vi "Comm_WriteRead.vi"(8 "error in (no error)":errorcluster, 9 "Code":string, 10 "Console In":string, 11 "Python":T1) -> (0 "error out":errorcluster, 2 "Console":string, 3 "Python":T1)   [LabVIEW 2022 SP3]
uses:
  PythonCtrl.ctl
  Processors.ctl
  <vilib>/Utility/error.llb/Trim Whitespace One-Sided.vi
panel:
  out "File sent":string[](array[string])
  out "Array":u32[](array[numeric])
  out "replies":string[](array[string])
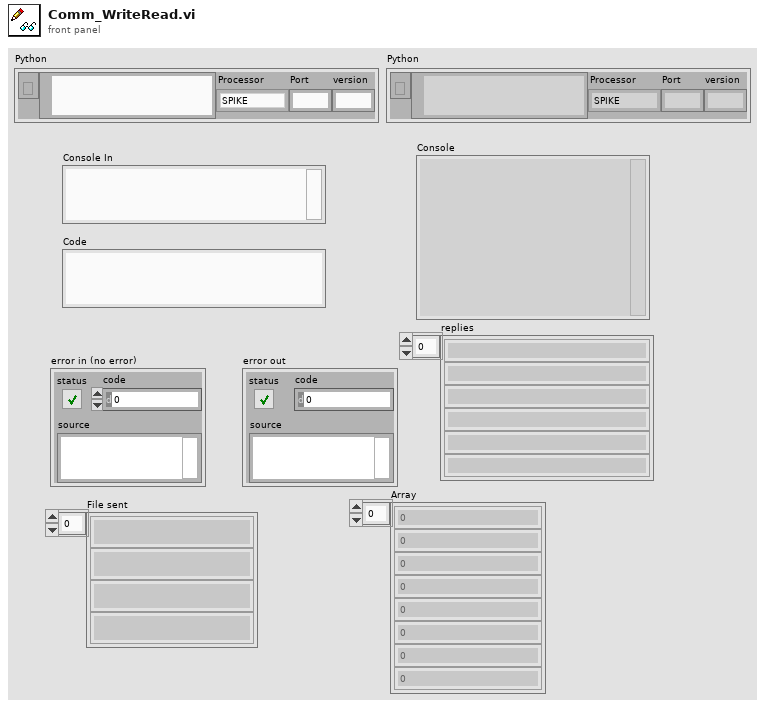
[diagram p1: front panel]
types:
  T1 = typedef "PythonCtrl.ctl" = cluster{"session":refnum<k35>, "PyPath":path, "Processor":T2, "Port":string, "version":string}
  T2 = typedef "Processors.ctl" = enum16{"SPIKE", "Pi", "Pi_ssh", "OpenMV", "Dunio"}
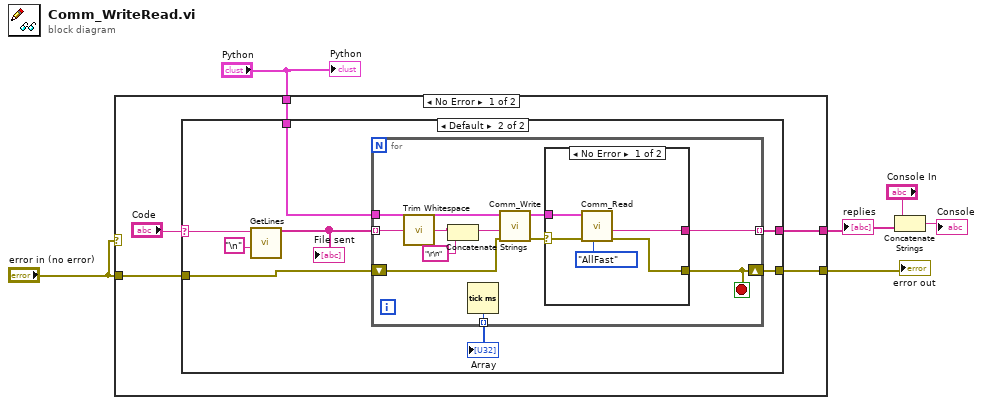
[diagram p0: block diagram]
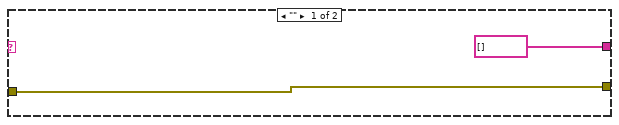
[diagram p2: hidden frame]
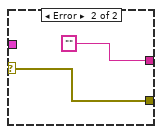
[diagram p3: hidden frame]
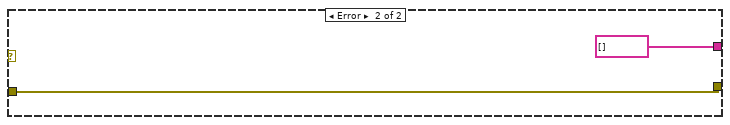
[diagram p4: hidden frame]
diagram:
  n1 = case shown="No Error" "error in (no error)" {
    tunnel: [w11 w40] -> w6
    tunnel: [w10 string[] []] -> w4
    tunnel: "Python" -> [w9 _]
    tunnel: "error in (no error)" -> [w7 w40]
    frame No Error {
      n2 = case shown="Default" "Code" {
        selector: "Code" -> [_ w15]
        tunnel: [w13 w21] -> w11
        tunnel: [string[] [] w20] -> w10
        tunnel: w9 -> [_ w19]
        tunnel: w7 -> [w13 w16]
        frame "" {
        }
        frame Default {
          n3 = call "GetLines.vi"("delimiter"="\n", "String"=w15) -> ("Array"=w18:string[])  [unwired: 9 in]
          "File sent" <- w18
          n4 = for {
            tunnel: w19 -> [w29]
            tunnel: w18 -> [w26] mode=indexing
            tunnel: [w28] -> w20 mode=indexing
            shift-right: [w27] -> w21
            shift-left: w16 -> [w31]
            tunnel: [w22] -> w17 mode=indexing
            stop <- w27 stop-if-true
            n5 = call <vilib>:"Trim Whitespace.vi"("string"=w26) -> ("trimmed string"=w24:string)  [unwired: 1 in]
            n6 = Concatenate Strings(w24, "\r\n" ("delimiter (Tab)")) -> (w25:string)
            n7 = Tick Count (ms)() -> (millisecond timer value=w22:u32)
            n8 = call "Comm_Write.vi"("error in (no error)"=w31, "Text to write"=w25, "Python"=w29) -> ("error out"=w30:errorcluster)  [unwired: 7 in, 1 out]
            n9 = case shown="No Error" w30 {
              selector: w30 -> [w34 w37]
              tunnel: [w36 w37] -> w27
              tunnel: [w32 ""] -> w28
              tunnel: w29 -> [w35 _]
              frame No Error {
                n10 = call "Comm_Read.vi"("Task"=enum16{"Instant", "All", "AllFast"}."AllFast", "error in (no error)"=w34, "Python"=w35) -> ("error out"=w36:errorcluster, "Text read"=w32:string)  [unwired: 7 in]
              }
              frame Error {
              }
            }
          }
          "Array" <- w17
        }
      }
    }
    frame Error {
    }
  }
  "error out" <- w6
  "replies" <- w4
  n11 = Concatenate Strings("Console In", w4) -> (→"Console":string)
  "Python" <- "Python"
